vi "Position Lat Lon Indicators.vi"(8 "Error In":errorcluster, 10 "Longitude":refnum<vi>, 11 "Latitude":refnum<vi>) -> (0 "Error Out":errorcluster)   [LabVIEW 2014]
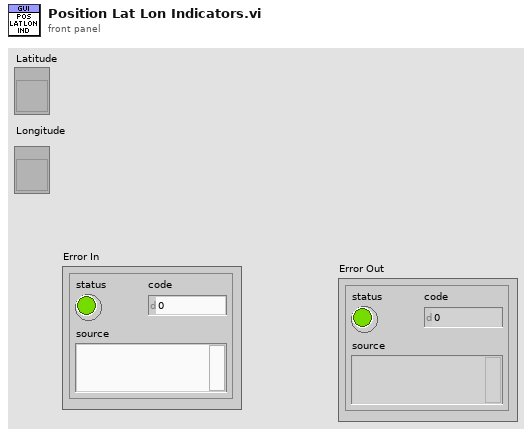
[diagram p1: front panel]
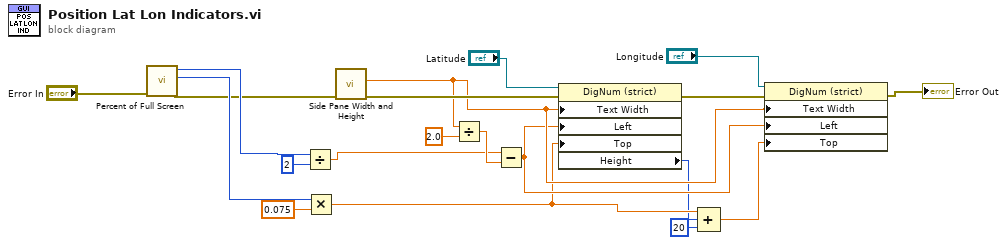
[diagram p0: block diagram]
diagram:
  n1 = call "Percent of Full Screen.vi"("error in (no error)"="Error In") -> ("error out"=w15:errorcluster, "Bottom"=w17:i16, "Right"=w19:i16)  [unwired: 8 in]
  n2 = Divide(x=w19, y=i16 2) -> (x/y=w11:dbl)
  n3 = Multiply(x=w17, y=0.075) -> (x*y=w4:dbl)
  n4 = call "Side Pane Width and Height.vi"("error in (no error)"=w15) -> ("error out"=w14:errorcluster, "Width"=w6:dbl)  [unwired: 8 in, 1 out]
  n5 = Divide(x=w6, y=2.0) -> (x/y=w12:dbl)
  n6 = Subtract(x=w11, y=w12) -> (x-y=w5:dbl)
  n7 = property class="DigNum (strict)"(reference="Latitude", error in=w14, "Text Width"=w6, "Left"=w5, "Top"=w4) -> (error out=w8:errorcluster, "Height"=w3:u32)  [unwired: 1 out]
  n8 = Compound Arithmetic op=ADD(w4, w3, u32 20 ("value")) -> (w1:dbl)
  n9 = property class="DigNum (strict)"(reference="Longitude", error in=w8, "Text Width"=w6, "Left"=w5, "Top"=w1) -> (error out=→"Error Out":errorcluster)  [unwired: 1 out]
